vi "New Game Board.vi"(6 "Color Box":u32(colorbox), 8 "error in (no error)":errorcluster, 10 "Grid Size":T1={"X"=45, "Y"=35}) -> (0 "error out":errorcluster, 3 "Game Board out":refnum<class "Game Board.lvclass">)   [LabVIEW 2020, in "Game Board.lvclass"]
uses:
  Game Board.lvclass
  Snake/Type Defs/Coordinates.ctl
  Game Board.lvclass/Game Board.ctl
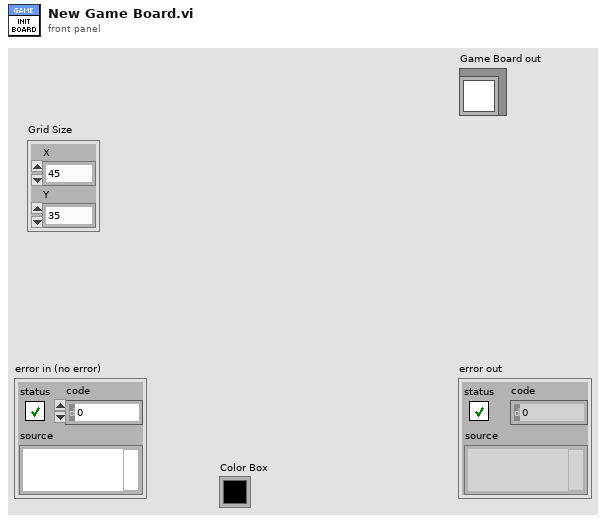
[diagram p1: front panel]
types:
  T1 = typedef "Coordinates.ctl" = cluster{"X":i32, "Y":i32}
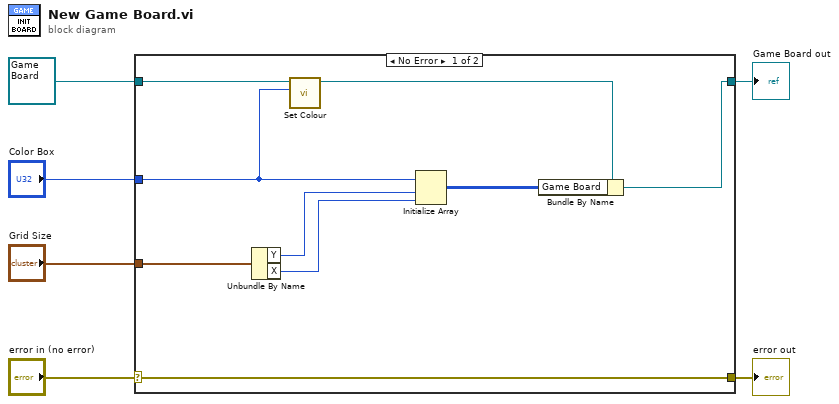
[diagram p0: block diagram]
diagram:
  n1 = case shown="No Error" "error in (no error)" {
    selector: "error in (no error)" -> [w15 w17]
    tunnel: [w15 w17] -> w5
    tunnel: [w13 w16] -> w3
    tunnel: refnum<class "Game Board.lvclass"> refnum ("Game Board in") -> [w11 w16]
    tunnel: "Color Box" -> [w12 _]
    tunnel: "Grid Size" -> [w9 _]
    frame No Error {
      n2 = Unbundle By Name(w9) -> ("Y"=w8:i32, "X"=w7:i32)
      n3 = call-dynamic "Set Colour.vi"("Componant Colour"=w12, "Game Componants in"=w11) -> ("Game Componants out"=w10:refnum<class "Game Board.lvclass">)  [unwired: 9 in]
      n4 = Initialize Array(w12, w8, w7) -> (w14:u32[][])
      n5 = Bundle By Name(cluster=w10, "Game Board"=w14) -> (w13:refnum<class "Game Board.lvclass">)
    }
    frame Error {
    }
  }
  "error out" <- w5
  "Game Board out" <- w3
